vi "SG Example.vi"() -> ()   [LabVIEW 2018]
uses:
  Source/SG/Typedefs/Waveform Timing Configuration.ctl
  Source/SG/Typedefs/PAEN Configuration.ctl
  <instrlib>/niRFSG/niRFSG.llb/niRFSG Exported Signal Destinations.ctl
  Source/SG/Typedefs/Instrument Configuration.ctl
  <instrlib>/niRFSG/niRFSG.llb/niRFSG Ref Clock Sources.ctl
  <instrlib>/niRFSG/niRFSG.llb/niRFSG Trigger Terminals.ctl
  Source/SG/SG.lvlib
panel:
  in  "Configurations":enum32{"General", "Dynamic Generation"}(tab)
  in  "resource name":refnum<k15>
  in  "Waveform File Path":path
  in  "Carrier Frequency (Hz)":dbl=1000000000.0 format="%#_6p"
  in  "DUT Average Input Power (dBm)":dbl=-20.0
  in  "External Attenuation (dB)":dbl
  in  "PAEN Configuration":T1={"PAEN Mode"=enum."Dynamic", "Command Enable Time (s)"=0.0, "Command Disable Time (s)"=0.0, "PA Enable Trigger Mode"=23001, "PA Enable Trigger Export Terminal"="PFI0"} {"PA Enable Trigger Mode" items=["Pulse"=23000, "Toggle"=23001]; "Command Disable Time (s)" format="%#_6p"; "Command Enable Time (s)" format="%#_6p"}
  in  "Waveform Timing Configuration":T3={"Duty Cycle (%)"=50.0, "Pre-Burst Time (s)"=1e-06, "Post-Burst Time (s)"=1e-06} {"Post-Burst Time (s)" format="%#_6p"; "Pre-Burst Time (s)" format="%#_6p"; "Duty Cycle (%)" min=1.0 max=100.0 step=1.0 format="%#_2d%%"}
  in  "stop":bool
  out "Status":string
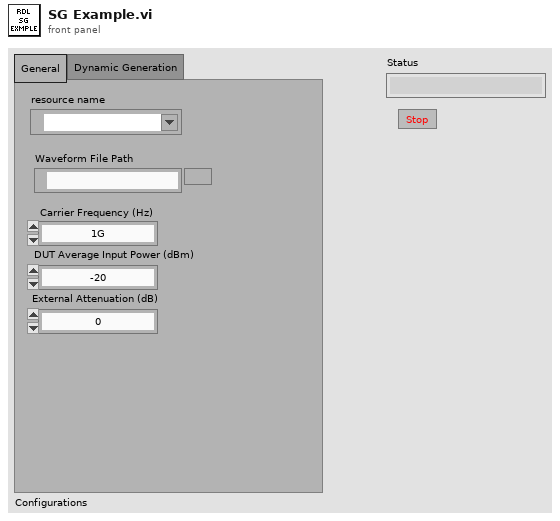
[diagram p1: front panel]
types:
  T1 = typedef "SG.lvlib/PAEN Configuration.ctl" = cluster{"PAEN Mode":enum16{"Disabled", "Static", "Dynamic"}, "Command Enable Time (s)":dbl, "Command Disable Time (s)":dbl, "PA Enable Trigger Mode":i32, "PA Enable Trigger Export Terminal":T2}
  T2 = typedef "niRFSG Exported Signal Destinations.ctl" = string
  T3 = typedef "SG.lvlib/Waveform Timing Configuration.ctl" = cluster{"Duty Cycle (%)":dbl, "Pre-Burst Time (s)":dbl, "Post-Burst Time (s)":dbl}
  T4 = typedef "SG.lvlib/Instrument Configuration.ctl" = cluster{"Reference Clock Source":T5, "Carrier Frequency (Hz)":dbl, "DUT Average Input Power (dBm)":dbl, "External Attenuation (dB)":dbl, "Marker 0 Export Terminal":T6, "Share LO  SG->SA":bool}
  T5 = typedef "niRFSG Ref Clock Sources.ctl" = string
  T6 = typedef "niRFSG Trigger Terminals.ctl" = string
  T7 = typedef "SG.lvlib/Waveform.ctl" = cluster{"Waveform Name":string, "Waveform":cluster{"x0":dbl, "dx":dbl, "y":csg[]}, "Signal Bandwidth (Hz)":dbl, "PAPR (dB)":dbl, "Burst Length (s)":dbl, "Sample Rate":dbl, "Burst Start Locations":i32[], "Burst Stop Locations":i32[], "Idle Duration Present?":bool}
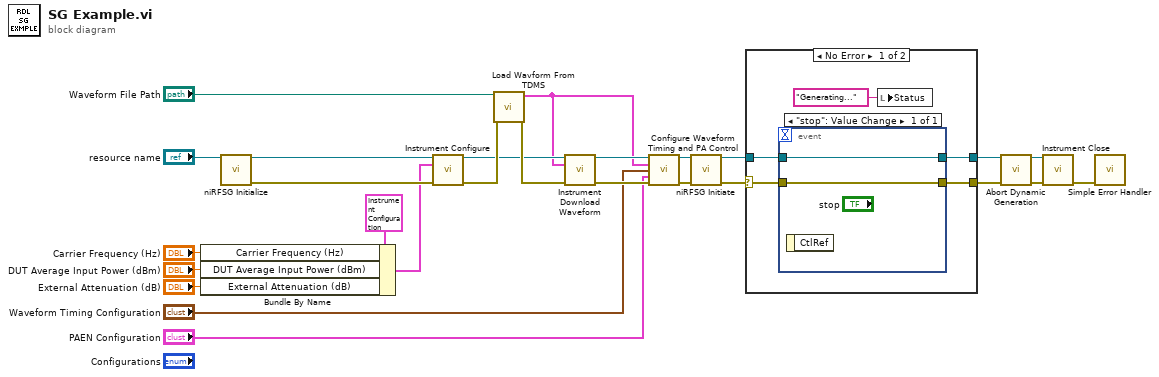
[diagram p0: block diagram]
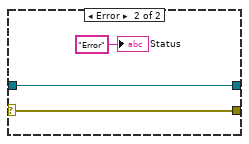
[diagram p2: hidden frame]
diagram:
  n1 = Bundle By Name(cluster=T4 {"Reference Clock Source"="OnboardClock", "Carrier Frequency (Hz)"=1000000000.0, "DUT Average Input Power (dBm)"=-20.0, "External Attenuation (dB)"=0.0, "Marker 0 Export Terminal"="", "Share LO  SG->SA"=FALSE} ("SG Configuration"), "Carrier Frequency (Hz)"="Carrier Frequency (Hz)", "DUT Average Input Power (dBm)"="DUT Average Input Power (dBm)", "External Attenuation (dB)"="External Attenuation (dB)") -> (w1:T4)
  n2 = call <instrlib>:"niRFSG Initialize.vi"("resource name"="resource name") -> ("instrument handle"=w20:refnum<k15>, "error out"=w26:errorcluster)  [unwired: 13 in]
  n3 = call "Instrument Configure.vi"("RFSG Session In"=w20, "SG Configuration"=w1, "error in (no error)"=w26) -> ("RFSG Session Out"=w17:refnum<k15>, "error out"=w22:errorcluster)  [unwired: 11 in]
  n4 = call "Load Wavform From TDMS.vi"("TDMS File Path"="Waveform File Path", "error in (no error)"=w22) -> ("Waveform"=w15:T7, "error out"=w21:errorcluster)  [unwired: 12 in]
  n5 = call "Instrument Download Waveform.vi"("RFSG handle"=w17, "Waveform In"=w15, "error in (no error)"=w21) -> ("RFSG handle out"=w16:refnum<k15>, "error out"=w23:errorcluster)  [unwired: 11 in]
  n6 = call "Configure Waveform Timing and PA Control.vi"("RFSG handle"=w16, "Waveform"=w15, "Waveform Timing Configuration"="Waveform Timing Configuration", "PAEN Configuration"="PAEN Configuration", "error in"=w23) -> ("RFSG handle out"=w19:refnum<k15>, "error out"=w25:errorcluster)  [unwired: 8 in, 1 out]
  n7 = call <instrlib>:"niRFSG Initiate.vi"("instrument handle"=w19, "error in"=w25) -> ("instrument handle out"=w12:refnum<k15>, "error out"=w7:errorcluster)  [unwired: 12 in]
  n8 = case shown="No Error" w7 {
    selector: w7 -> [w27 w36]
    tunnel: w12 -> [w31 w35]
    tunnel: [w30 w35] -> w11
    tunnel: [w29 w36] -> w10
    frame No Error {
      n9 = event shown="[0] \"stop\": Value Change" {
        selector: _ -> [_]
        dyn-events: _ -> [_]
        timeout: _ -> [_]
        tunnel: w27 -> [w32]
        tunnel: w31 -> [w33]
        tunnel: [w33] -> w30
        tunnel: [w32] -> w29
        event "stop": Value Change {
          n10 = event-data() -> ()  [unwired: 1 in, 1 out]
        }
      }
      n11 = local write "Status"("Generating..." ("Status")) -> ()
    }
    frame Error {
      "Status" <- "Error" ("Status")
    }
  }
  n12 = call "Abort Dynamic Generation.vi"("RFSG handle"=w11, "error in (no error)"=w10) -> ("RFSG handle out"=w18:refnum<k15>, "error out"=w24:errorcluster)  [unwired: 12 in]
  n13 = call "Instrument Close.vi"("RFSG Handle"=w18, "error in (no error)"=w24) -> ("error out"=w9:errorcluster)  [unwired: 13 in]
  n14 = call <vilib>:"Simple Error Handler.vi"("error in (no error)"=w9) -> ()  [unwired: 4 in, 5 out]
